vi "P2PSendData.vi"(8 "error in (no error)":errorcluster, 9 "DataExchange":T1, 10 "TargetDeviceEnqueuer":refnum<class "Message Enqueuer.lvclass">, 11 "GRMActor in":refnum<class "GeneralRMActor.lvclass">) -> (0 "error out":errorcluster, 3 "GRMActor out":refnum<class "GeneralRMActor.lvclass">)   [LabVIEW 2020, in "GeneralRMActor.lvlib" / "GeneralRMActor.lvclass"]
uses:
  GeneralRMActor.lvclass
  Device/Device/DataExchange.ctl
  <vilib>/ActorFramework/Message Enqueuer/Message Enqueuer.lvclass
  Interface/DataListener Messages/OnDataChange Msg/OnDataChange Msg.lvclass/OnDataChange Msg.ctl
  <vilib>/ActorFramework/Message Enqueuer/Message Enqueuer.lvclass/Message Enqueuer.ctl
  <vilib>/ActorFramework/Message Enqueuer/Enqueue.vi
  Interface/DataListener Messages/OnDataChange Msg/OnDataChange Msg.lvclass
  C:/Program Files/National Instruments/LabVIEW 2020/vi.lib/ActorFramework/Message/Message.lvclass
  <vilib>/ActorFramework/Message Priority Queue/Priority Enqueue.vi
  Interface/DataListener/DataListener.lvclass
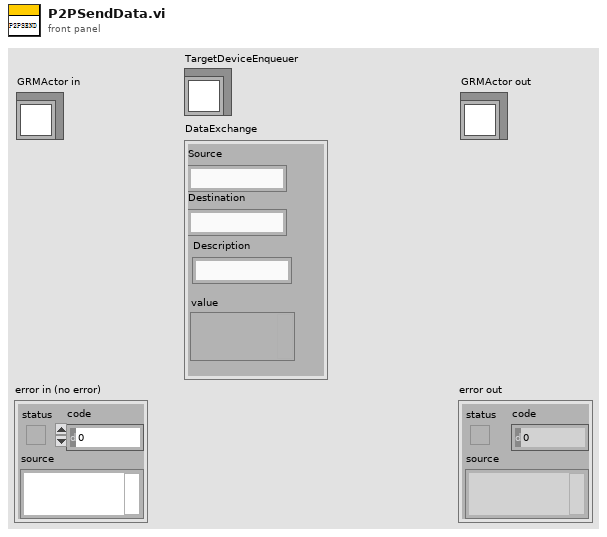
[diagram p1: front panel]
types:
  T1 = typedef "DataListener.lvclass/DataExchange.ctl" = cluster{"Source":string, "Destination":string, "Description":string, "value":variant}
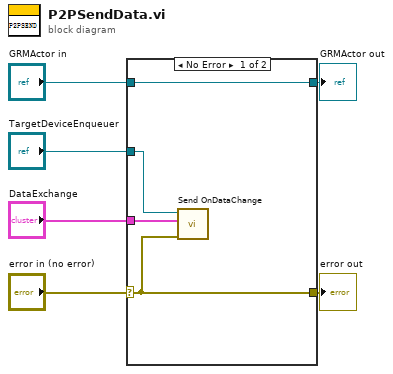
[diagram p0: block diagram]
diagram:
  n1 = case shown="No Error" "error in (no error)" {
    selector: "error in (no error)" -> [w7 w12]
    tunnel: [w7 w12] -> w1
    tunnel: [w10 w11] -> w3
    tunnel: "GRMActor in" -> [w10 w11]
    tunnel: "DataExchange" -> [w9 _]
    tunnel: "TargetDeviceEnqueuer" -> [w8 _]
    frame No Error {
      n2 = call "Send OnDataChange.vi"("error in (no error)"=w7, "DataExchange"=w9, "Message Enqueuer"=w8) -> ()  [unwired: 7 in, 2 out]
    }
    frame Error {
    }
  }
  "error out" <- w1
  "GRMActor out" <- w3
